vi "DataTreeOrderScan.vi"(8 "error in (no error)":errorcluster, 9 "Scan":i32, 10 "SessIndex":i32, 11 "Scans":cluster{i32[]}[](array[cluster])) -> (0 "error out":errorcluster, 1 "ScanIndex":i32, 3 "Scans Out":cluster{i32[]}[](array[cluster]))   [LabVIEW 2019]
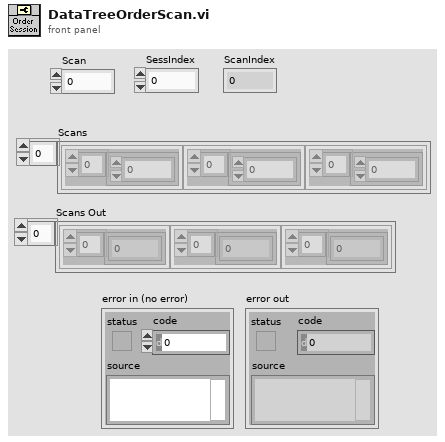
[diagram p1: front panel]
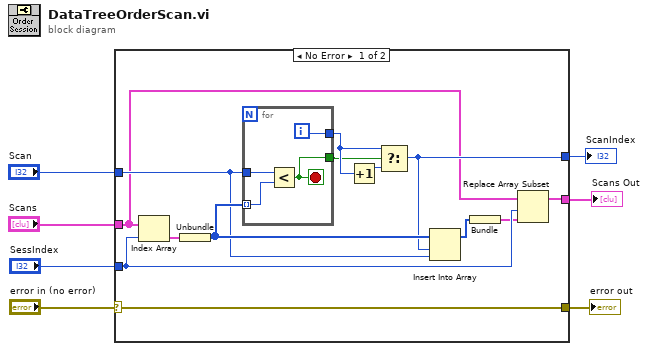
[diagram p0: block diagram]
diagram:
  n1 = case shown="No Error" "error in (no error)" {
    selector: "error in (no error)" -> [w20 w25]
    tunnel: [w20 w25] -> w6
    tunnel: "Scans" -> [w12 _]
    tunnel: "Scan" -> [w14 _]
    tunnel: [w10 _] -> w3
    tunnel: "SessIndex" -> [w11 _]
    tunnel: [w13 _] -> w1
    frame No Error {
      n2 = Index Array(array=w12, index=w11) -> (element=w19:cluster{i32[]})
      n3 = Unbundle(w19) -> (w15:i32[])
      n4 = for {
        tunnel: w15 -> [w23] mode=indexing
        tunnel: w14 -> [w24]
        tunnel: [w22] -> w17
        tunnel: [w21] -> w16
        i -> [w22]
        stop <- w21 stop-if-true
        n5 = Less?(x=w24, y=w23) -> (x < y?=w21:bool)
      }
      n6 = Increment(x=w17) -> (x+1=w18:i32)
      n7 = Select(t=w17, s=w16, f=w18) -> (s? t:f=w13:i32)
      n8 = Insert Into Array(array=w15, index=w13, new element=w14) -> (w9:i32[])
      n9 = Bundle(w9) -> (w8:cluster{i32[]})  [unwired: 1 in]
      n10 = Replace Array Subset(array=w12, new element=w8, index=w11) -> (w10:cluster{i32[]}[])
    }
    frame Error {
    }
  }
  "error out" <- w6
  "Scans Out" <- w3
  "ScanIndex" <- w1
